vi "Push Points Batch_YX.vi"(8 "error in (no error)":errorcluster, 10 "Points":cluster{"Value":dbl, "Time Stamp":timestamp}[](array[cluster]) {"Time Stamp" format="%<%x %.3X>T"}, 11 "Channel in":refnum<class "Channel.lvclass">) -> (0 "error out":errorcluster, 3 "Channel out":refnum<class "Channel.lvclass">)   [LabVIEW 2020, in "Nominal Streaming.lvlib" / "Channel.lvclass"]
doc: "Pushes point data to Nominal Core.\nData can be presented in either [{timestamp, value}] or [{value, timestamp}].\nAny `Not a Number` (NaN) values will be filtered out.\nReturns an error if there is a mismatch in input array sizes."
uses:
  Channel.lvclass
  Channel.lvclass/Channel.ctl
  <vilib>/LabVIEW Open Source Project/Epoch Date & Time/epoch.UNIX/Epoch.UNIX.lvclass
  C:/Program Files/National Instruments/LabVIEW 2020/vi.lib/LabVIEW Open Source Project/Epoch Date & Time/epoch/Epoch.lvclass
  <vilib>/LabVIEW Open Source Project/Epoch Date & Time/Get Epoch Time.vi
  Stream/Stream.lvclass
  Nominal Streaming/Nominal Streaming.lvlib
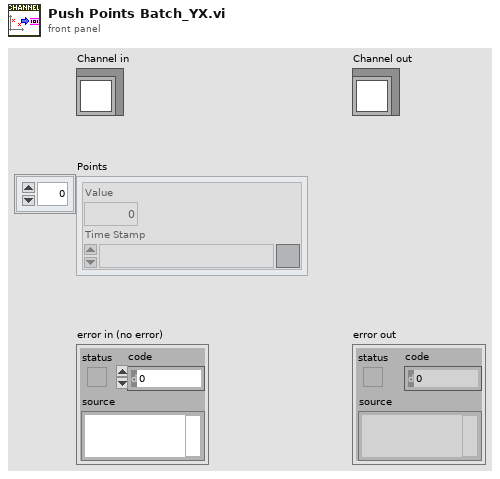
[diagram p1: front panel]
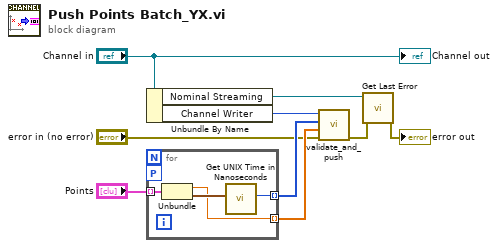
[diagram p0: block diagram]
diagram:
  n1 = Unbundle By Name("Channel in") -> ("Nominal Streaming"=w7:refnum<class "Stream.lvclass">, "Channel Writer"=w5:u64)
  n2 = for {
    tunnel: "Points" -> [w12] mode=indexing
    tunnel: [w13] -> w4 mode=indexing
    tunnel: [w10] -> w3 mode=indexing
    workers-P: _ -> [_]
    n3 = Unbundle(w12) -> ("Value"=w10:dbl, "Time Stamp"=w11:timestamp)
    n4 = call "Get UNIX Time in Nanoseconds.vi"("Time Stamp"=w11) -> ("UNIX Time (ns)"=w13:u64)  [unwired: 10 in]
  }
  n5 = call "validate_and_push.vi"("error in (no error)"="error in (no error)", "values"=w3, "timestamps_ns"=w4, "writer_handle"=w5) -> ("error out"=w1:errorcluster)  [unwired: 7 in]
  n6 = call "Get Last Error.vi"("error in (no error)"=w1, "Nominal Streaming in"=w7) -> ("error out"=→"error out":errorcluster)  [unwired: 8 in, 1 out]
  "Channel out" <- "Channel in"
